vi "Get XTAL Frequency.vi"(8 "error in (no error)":errorcluster, 11 "DeviceRefnum":u64) -> (0 "error out":errorcluster, 1 "Tuner Frequency":dbl, 2 "RTL Frequency":dbl, 3 "DeviceRefnum Out":u64)   [LabVIEW 2016]
doc: "Get crystal oscillator frequencies used for the RTL2832 and the tuner IC."
panel:
  in  "tuner_freq":u32
  in  "rtl_freq":u32
  out "function return":i32
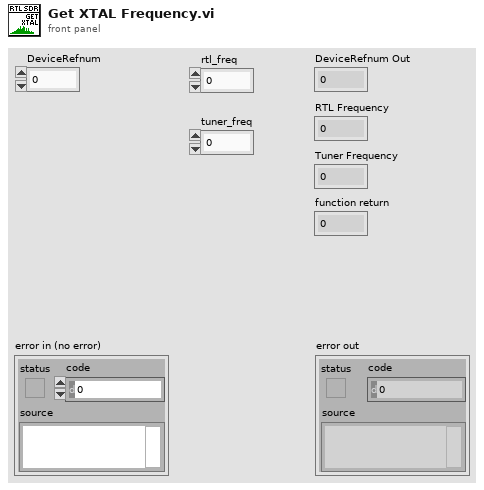
[diagram p1: front panel]
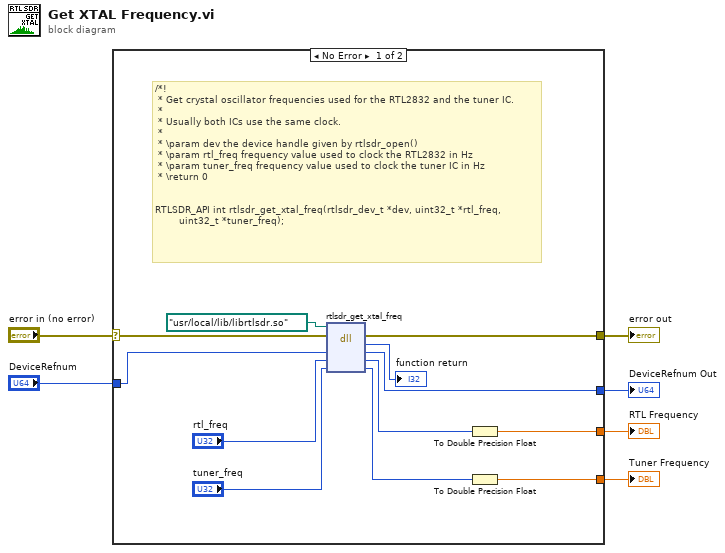
[diagram p0: block diagram]
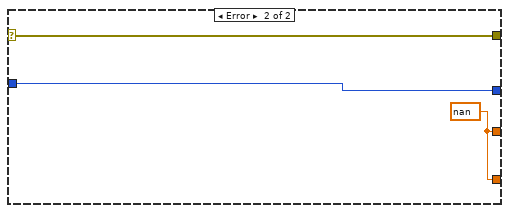
[diagram p2: hidden frame]
diagram:
  n1 = case shown="No Error" "error in (no error)" {
    selector: "error in (no error)" -> [w10 w21]
    tunnel: "DeviceRefnum" -> [w14 w20]
    tunnel: [w15 w21] -> w4
    tunnel: [w9 w20] -> w3
    tunnel: [w8 w19] -> w2
    tunnel: [w7 w19] -> w1
    frame No Error {
      # "/*!\n * Get crystal oscillator frequencies used for the RTL2832 and the tuner IC.\n *\n * Usually both ICs use the same clock.\n *\n * \\param dev the device handle given by rtlsdr_open()\n * \\param rtl_freq frequency value used to clock the RTL2832 in Hz\n * \\param tuner_freq frequency value used to clock the tuner IC in Hz\n * \\return 0 \n\n\nRTLSDR_API int rtlsdr_get_xtal_freq(rtlsdr_dev_t *dev, uint32_t *rtl_freq,\n\t\t\t\t    uint32_t *tuner_freq);"
      n2 = dll-call lib="C:/Program Files (x86)/National Instruments/LabVIEW 2016/user.lib/rtlsdr/rtlsdr.*" fn="rtlsdr_get_xtal_freq"(path in=path "/usr/local/lib/librtlsdr.so", error in=w10, "DeviceRefnum"=w14, "rtl_freq"="rtl_freq", "tuner_freq"="tuner_freq") -> (error out=w15:errorcluster, "return type"=→"function return":i32, "DeviceRefnum"=w9:u64, "rtl_freq"=w12:u32, "tuner_freq"=w11:u32)  [unwired: 1 in, 1 out]
      n3 = To Double Precision Float(number=w12) -> (double precision float=w8:dbl)
      n4 = To Double Precision Float(number=w11) -> (double precision float=w7:dbl)
    }
    frame Error {
      w19 = nan
    }
  }
  "error out" <- w4
  "DeviceRefnum Out" <- w3
  "RTL Frequency" <- w2
  "Tuner Frequency" <- w1
